vi "Read Image.vi"() -> ()   [LabVIEW 2014]
doc: "This demo reads a file and displays it."
uses:
  MSC Image_class/MSC Image.lvclass
panel:
  in  "path":path=path "Browse for Path ->"
  out "error out":errorcluster
  out "picture":picture
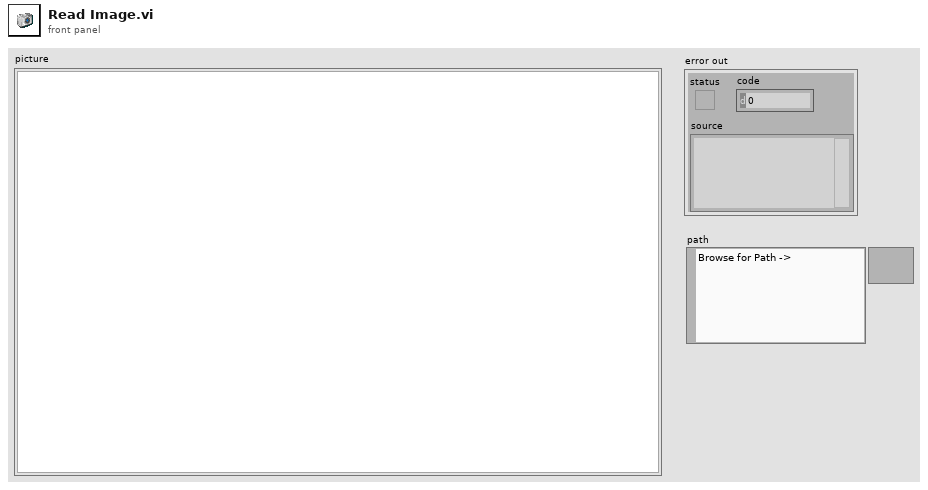
[diagram p1: front panel]
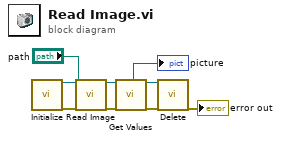
[diagram p0: block diagram]
diagram:
  n1 = call "Initialize.vi"() -> ("image out"=w5:refnum<class "MSC Image.lvclass">, "error out"=w4:errorcluster)  [unwired: 18 in]
  n2 = call-dynamic "Read Image.vi"("image in"=w5, "image path"="path", "error in (no error)"=w4) -> ("image out"=w2:refnum<class "MSC Image.lvclass">, "error out"=w3:errorcluster)  [unwired: 15 in]
  n3 = call-dynamic "Get Values.vi"("image in"=w2, "error in (no error)"=w3) -> ("picture"=→"picture":picture, "image out"=w8:refnum<class "MSC Image.lvclass">, "error out"=w7:errorcluster)  [unwired: 10 in, 5 out]
  n4 = call-dynamic "Delete.vi"("image in"=w8, "error in (no error)"=w7) -> ("error out"=→"error out":errorcluster)  [unwired: 17 in]
